vi "Autonomous Independent.vi"() -> ()   [LabVIEW 2016]
doc: "This VI is called when autonomous begins, and will automatically be terminated when autonomous ends. You can carry out timed or sensor driven robot movement independently without needing to return to the caller."
uses:
  <vilib>/Rock Robotics/WPI/ThirdParty/CanMotor/TalonSRX/WPI_CANTalonSRX_APIControlMode.ctl
  <vilib>/Rock Robotics/WPI/DriverStation/WPI_DriverStationAllianceInfo.ctl
  <vilib>/Rock Robotics/Network Tables/NT Read Boolean.vi
  Robot Global Data.vi
panel:
  out "Auto time":u32
  # "Be sure to right-click and choose Data Operations>>Make Current Value default if you want to save the array values with the VI"
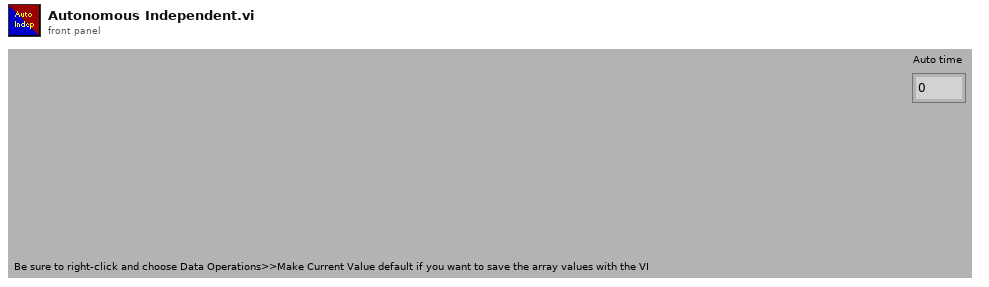
[diagram p1: front panel]
types:
  T1 = typedef "WPI_DriverStationAllianceInfo.ctl" = enum16{"Red", "Blue", "Invalid"}
  T2 = typedef "WPI_CANTalonSRX_APIControlMode.ctl" = enum8{"Percent VBus", "Speed", "Position", "Slave", "Unchanged / Invalid", "Voltage Compensation", "Current", "Motion Profile", "Motion Magic"}
  T3 = typedef "WPI_MotorControlDeviceRef.ctl" = cluster{"DeviceStatus":errorcluster, "Type":T4, "PWM":cluster{"PWM Channel":T5, "DeadBand":T6}, "CAN":cluster{"Device Number":u8, "SetOutput VI Ref":variant, "GetOutput VI Ref":variant, "Enable VI Ref":variant, "Disable VI Ref":variant, "Data":variant}, "Invert":bool}
  T4 = typedef "WPI_MotorControlType.ctl" = enum16{"PWM", "CAN"}
  T5 = typedef "FPGA_DIOPWMChannel.ctl" = enum8{"PWM 0", "PWM 1", "PWM 2", "PWM 3", "PWM 4", "PWM 5", "PWM 6", "PWM 7", "PWM 8", "PWM 9", "PWM MXP 0", "PWM MXP 1", "PWM MXP 2", "PWM MXP 3", "PWM MXP 4", "PWM MXP 5", "PWM MXP 6", "PWM MXP 7", "PWM MXP 8", "PWM MXP 9", "Invalid"}
  T6 = typedef "WPI_PWMDeadband.ctl" = cluster{"Name":string, "maxPositivePwm":i32, "minPositivePwm":i32, "centerPwm":i32, "maxNegativePwm":i32, "minNegativePwm":i32, "angularRange":u16}
  T7 = cluster{"Yaw":dbl, "Roll":dbl, "Pitch":dbl, "Heading":dbl, "Fused Heading":dbl}
  T8 = typedef "WPI_CANTalonSRX_GlobalStatus.ctl" = cluster{"Applied Throttle":dbl, "Module Enabled":bool, "CAN Error":errorcluster, "Closed Loop Error":dbl, "Forward Limit Switch Closed":bool, "Reverse Limit Switch Closed":bool, "Sensor Position":dbl, "Sensor Velocity":dbl, "Current":dbl, "Sticky Fault - Over Temp":bool, "Sticky Fault - Under Voltage":bool, "Sticky Fault - Forward Limit":bool, "Sticky Fault - Reverse Limit":bool, "Sticky Fault - Forward Soft Limit":bool, "Sticky Fault - Reverse Soft Limit":bool, "Brake is Enabled":bool, "Encoder Position":dbl, "Encoder Velocity":dbl, "Encoder Index Count":dbl, "Encoder A Pin State":bool, "Encoder B Pin State":bool, "Encoder Index Pin State":bool, "Analog In":dbl, "Analog In Velocity":dbl, "Temperature (C)":dbl, "Battery Voltage":dbl, "Control 5 Is Supported":bool, "Current Profile Slot Select":dbl, "Pos Div 8":bool, "Vel Div 4":bool, "Pulse Width Position":i32, "Pulse Width Velocity":i32, "Pulse Width Rise To Rise (us)":i32, "Pulse Width Rise To Fall (us)":i32, "Mot Prof Active Is Under Run":bool, "Mot Prof Active Has Under Run":bool, "Mot Prof Active Is Last":bool, "Mot Prof Active Velocity Only":bool, "Mot Prof Active Is Valid":bool, "Mot Prof Buffer Is Full":bool, "Mot Prof Active Profile Slot Select":i32, "Mot Prof NextID":i32, "Mot Prof Count":i32, "Mot Prof Active Velocity":dbl, "Mot Prof Active Position":dbl, "Mot Prof Output Enable":i32}
  T9 = cluster{"proportional gain (Kc)":dbl, "integral time (Ti, min)":dbl, "derivative time (Td, min)":dbl}
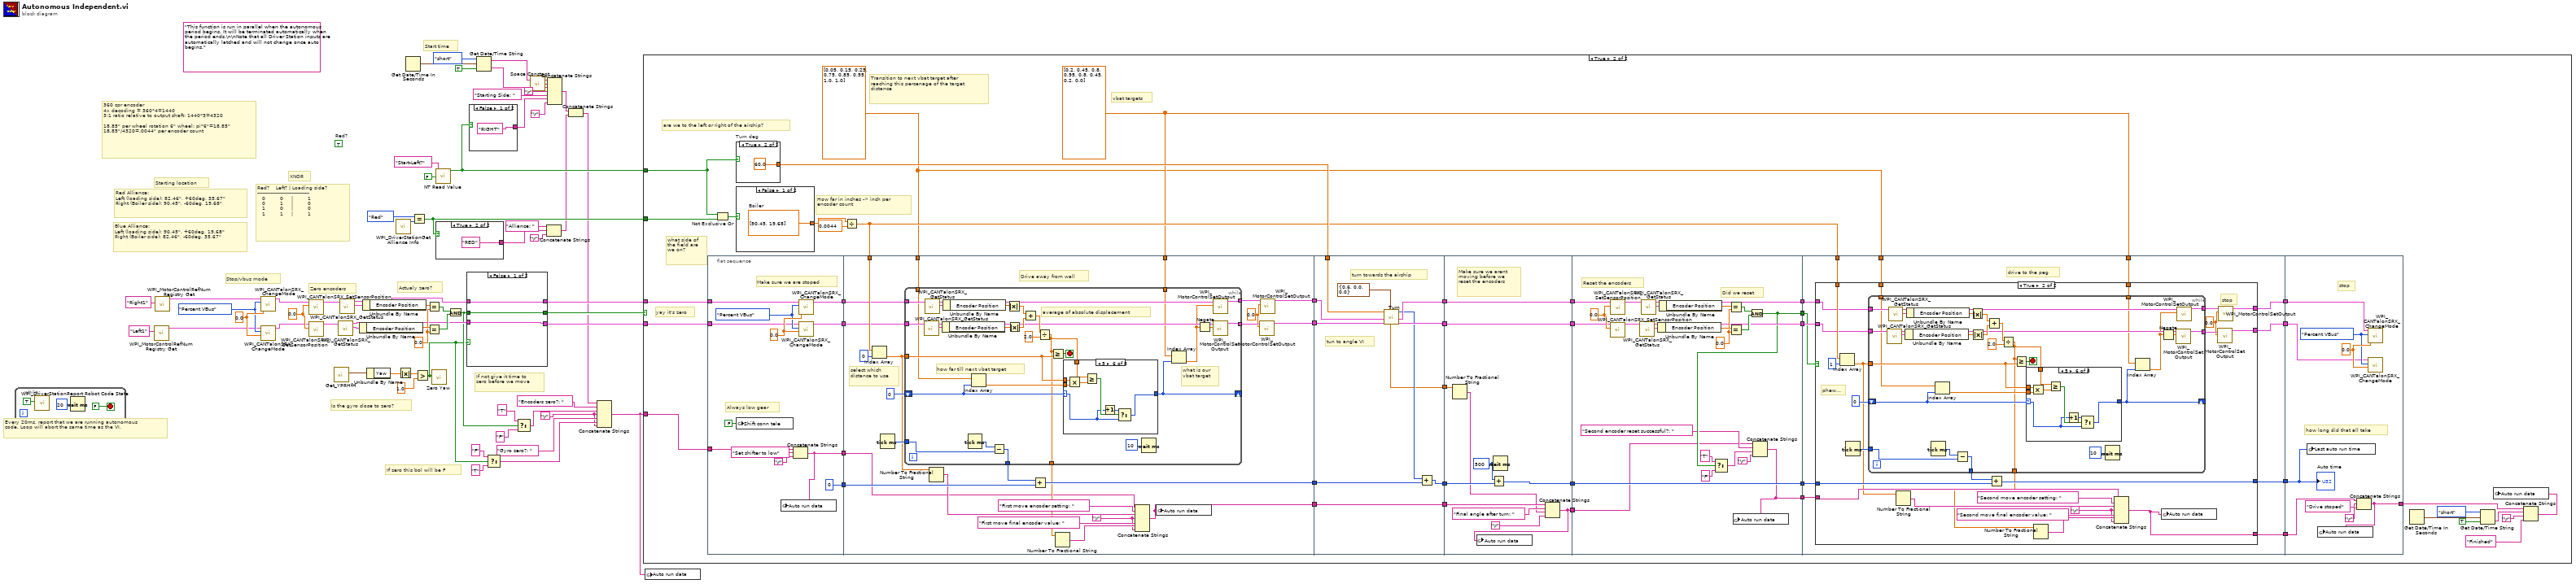
[diagram p0: block diagram]
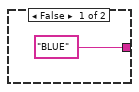
[diagram p2: hidden frame]
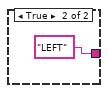
[diagram p3: hidden frame]
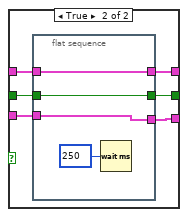
[diagram p4: hidden frame]
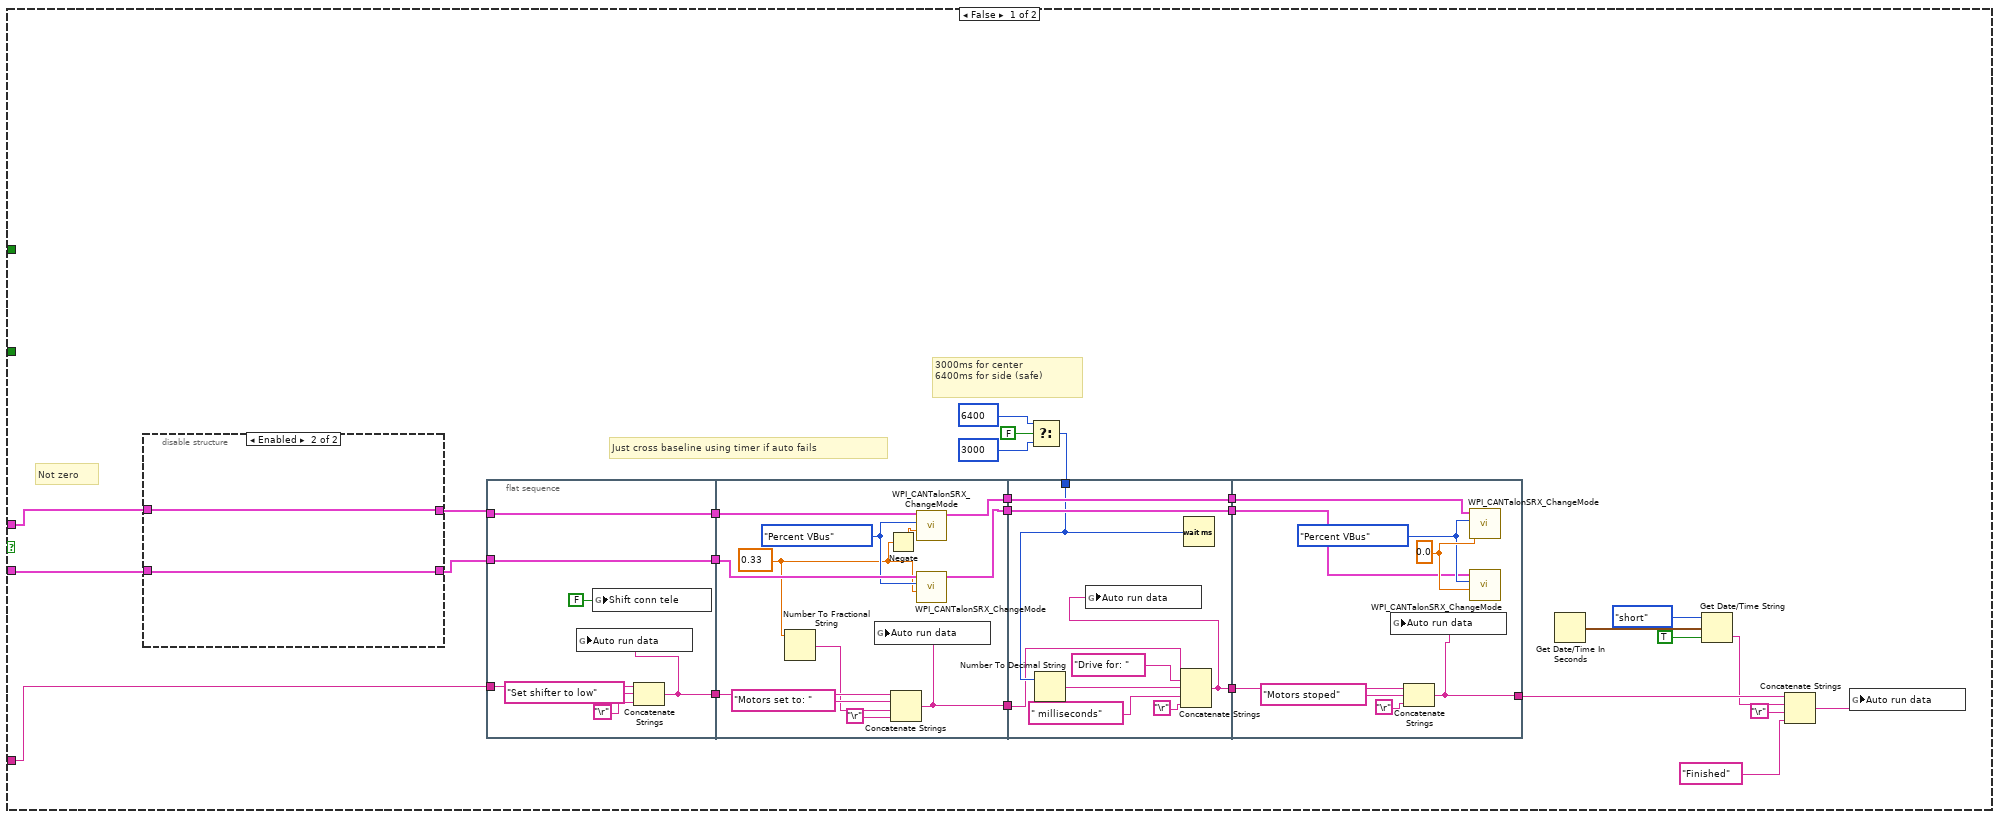
[diagram p5: hidden frame]
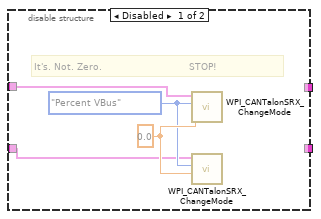
[diagram p6: hidden frame]
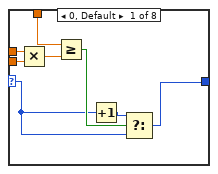
[diagram p7: hidden frame]
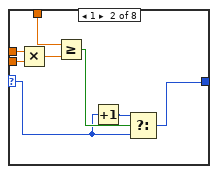
[diagram p8: hidden frame]
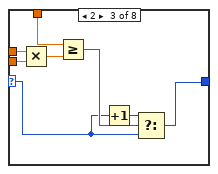
[diagram p9: hidden frame]
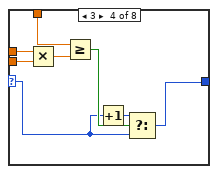
[diagram p10: hidden frame]
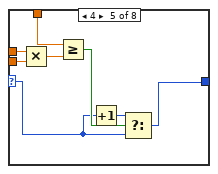
[diagram p11: hidden frame]
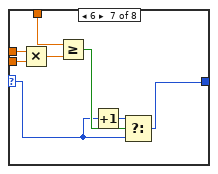
[diagram p12: hidden frame]
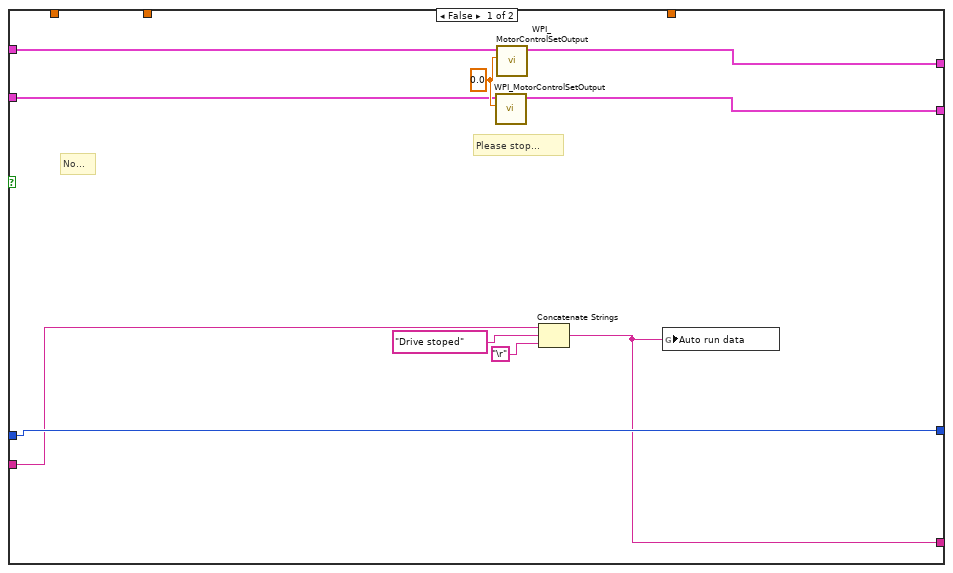
[diagram p14: hidden frame]
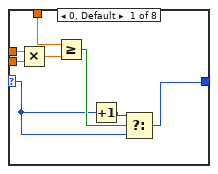
[diagram p15: hidden frame]
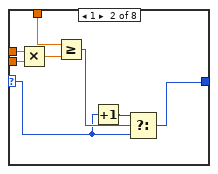
[diagram p16: hidden frame]
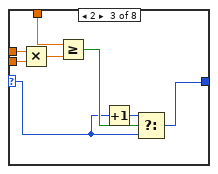
[diagram p17: hidden frame]
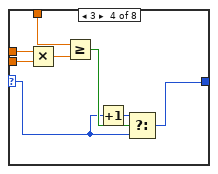
[diagram p18: hidden frame]
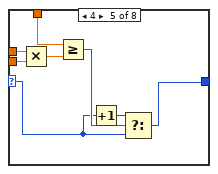
[diagram p19: hidden frame]
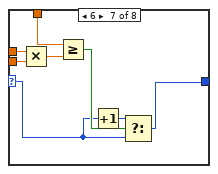
[diagram p20: hidden frame]
diagram:
  w9 = "\r"
  w40 = WPI_CANTalonSRX_APIControlMode."Percent VBus" ("Control Mode")
  w41 = 0.0
  w52 = 0.0
  w59 = 0.0 ("New Sensor Position")
  (unwired) TRUE  # Red?
  (unwired) "This function is run in parallel when the autonomous period begins. It will be terminated automatically when the period ends.\n\nNote that all Driver Station inputs are automatically latched and will not change once auto begins."
  # "Start time"
  # "If zero this bol will be F"
  # "Starting location"
  # "If not give it time to\nzero before we move"
  # "Is the gyro close to zero?"
  # "Stop/vbus mode"
  # "Zero encoders"
  # "Actualy zero?"
  # "XNOR"
  # "Red?    Left? | Loading side?\n--------------------------------\n   0         0     |         1        \n   0         1     |         0\n   1         0     |         0\n   1         1     |         1"
  # "Blue Alliance:\nLeft (loading side): 90.45\", +60deg, 19.68\"\nRight (Boiler side): 82.46\", -60deg, 35.67\""
  # "Red Alliance:\nLeft (loading side): 82.46\", +60deg, 35.67\"\nRight (Boiler side): 90.45\", -60deg, 19.68\""
  # "360 cpr encoder\n4x decoding = 360*4=1440\n3:1 ratio relative to output shaft: 1440*3=4320\n\n18.85\" per wheel rotation 6\" wheel: pi*6\"=18.85\"\n18.85\"/4320=.0044\" per encoder count"
  # "Every 20ms, report that we are running autonomous\ncode. Loop will abort the same time as the VI."
  n1 = while {
    stop <- FALSE stop-if-true
    n2 = call <vilib>:"WPI_DriverStationReport Robot Code State.vi"("Autonomous"=TRUE) -> ()  [unwired: 10 in, 1 out]
    n3 = Wait (ms)(milliseconds to wait=u32 20) -> ()  [unwired: 1 out]
  }
  n4 = call <vilib>:"WPI_MotorControlRefNum Registry Get.vi"("refnum name"="Left1") -> ("MotorControlDevRef"=w38:T3)  [unwired: 9 in, 1 out]
  n5 = call <vilib>:"WPI_MotorControlRefNum Registry Get.vi"("refnum name"="Right1") -> ("MotorControlDevRef"=w39:T3)  [unwired: 9 in, 1 out]
  n6 = call <vilib>:"WPI_CANTalonSRX_ChangeMode.vi"("Output"=w41, "Control Mode"=w40, "CAN Talon SRX Ref"=w39) -> ("CAN Talon SRX Ref"=w37:T3)  [unwired: 7 in, 1 out]
  n7 = call <vilib>:"WPI_CANTalonSRX_ChangeMode.vi"("Output"=w41, "Control Mode"=w40, "CAN Talon SRX Ref"=w38) -> ("CAN Talon SRX Ref"=w36:T3)  [unwired: 7 in, 1 out]
  n8 = call <vilib>:"WPI_CANTalonSRX_SetSensorPosition.vi"("New Sensor Position"=w59, "CAN Talon SRX Ref"=w36) -> ("CAN Talon SRX Ref"=w55:T3)  [unwired: 8 in, 1 out]
  n9 = call <vilib>:"WPI_CANTalonSRX_SetSensorPosition.vi"("New Sensor Position"=w59, "CAN Talon SRX Ref"=w37) -> ("CAN Talon SRX Ref"=w56:T3)  [unwired: 8 in, 1 out]
  n10 = call <vilib>:"Get_YPRHfH.vi"() -> ("YRPHfH"=w49:T7)  [unwired: 11 in]
  n11 = call <vilib>:"WPI_CANTalonSRX_GetStatus.vi"("CAN Talon SRX Ref"=w55) -> ("Talon SRX Status"=w57:T8, "CAN Talon SRX Ref"=w42:T3)  [unwired: 8 in, 1 out]
  n12 = call <vilib>:"WPI_CANTalonSRX_GetStatus.vi"("CAN Talon SRX Ref"=w56) -> ("Talon SRX Status"=w58:T8, "CAN Talon SRX Ref"=w43:T3)  [unwired: 8 in, 1 out]
  n13 = Unbundle By Name(w57) -> ("Encoder Position"=w53:dbl)
  n14 = Unbundle By Name(w58) -> ("Encoder Position"=w54:dbl)
  n15 = Unbundle By Name(w49) -> ("Yaw"=w48:dbl)
  n16 = call <vilib>:"WPI_DriverStationGet Alliance Info.vi"() -> ("Alliance"=w25:T1)  [unwired: 11 out]
  n17 = Absolute Value(x=w48) -> (abs(x)=w33:dbl)
  n18 = Get Date/Time In Seconds() -> (seconds since 1Jan1904=w7:timestamp)
  n19 = Equal?(x=WPI_DriverStationAllianceInfo."Red" ("Alliance"), y=w25) -> (x = y?=w23:bool)
  n20 = Greater?(x=w33, y=1.0) -> (0:w29:bool)
  n21 = Equal?(x=w54, y=w52) -> (x = y?=w51:bool)
  n22 = Equal?(x=w53, y=w52) -> (x = y?=w50:bool)
  n23 = call <vilib>:"Zero Yaw.vi"("Zero"=w29) -> ()  [unwired: 11 in]
  n24 = call-poly <vilib>:"NT Read Value.vi"("Default Value"=FALSE, "Name"="Start-Left?") -> ("Boolean"=w24:bool)  [unwired: 8 in, 1 out]
  n25 = case shown="True" w23 {
    tunnel: ["BLUE" "RED"] -> w21
    frame False {
    }
    frame True {
    }
  }
  n26 = And(x=w51, y=w50) -> (x .and. y?=w30:bool)
  n27 = case shown="False" w29 {
    tunnel: [w68 w75] -> w46
    tunnel: [w67 w71] -> w45
    tunnel: w30 -> [w69 w72]
    tunnel: [w69 w73] -> w44
    tunnel: w43 -> [w68 w74]
    tunnel: w42 -> [w67 w70]
    frame False {
    }
    frame True {
      n28 = flat-sequence {
        tunnel: [w79] -> w75
        tunnel: w74 -> [w79]
        tunnel: [w78] -> w73
        tunnel: w72 -> [w78]
        tunnel: [w77] -> w71
        tunnel: w70 -> [w77]
        frame #0 {
          n29 = Wait (ms)(milliseconds to wait=u32 250) -> ()  [unwired: 1 out]
        }
      }
    }
  }
  n30 = case shown="False" w24 {
    tunnel: ["RIGHT" "LEFT"] -> w17
    frame False {
    }
    frame True {
    }
  }
  n31 = Get Date/Time String(date format (0)=enum16{"short", "long", "abbreviated"}."short", seconds (now)=w7, want seconds? (F)=TRUE) -> (date string=w3:string, time string=w2:string)
  n32 = Select(t="F", s=w29, f="T") -> (s? t:f=w10:string)
  n33 = Select(t="T", s=w30, f="F") -> (s? t:f=w12:string)
  n34 = call <vilib>:"Space Constant.vi"() -> ("String"=w1:string)
  n35 = Concatenate Strings("Alliance: ", w21, "\r") -> (w15:string)
  n36 = Concatenate Strings(w3, w1, w2, "\r", "Starting Side: ", w17, "\r") -> (w16:string)
  n37 = Concatenate Strings(w16, w15) -> (w14:string)
  n38 = Concatenate Strings(w14, "Encoders zero?: ", w12, w9, "Gyro zero?: ", w10, w9) -> (w8:string)
  n39 = case shown="True" w44 {
    tunnel: w46 -> [w107 w181]
    tunnel: w45 -> [w106 w180]
    tunnel: w24 -> [_ w167]
    tunnel: w23 -> [_ w166]
    tunnel: w8 -> [w97 w165]
    frame False {
      # "3000ms for center\n6400ms for side (safe)"
      # "Not zero"
      # "Just cross baseline using timer if auto fails"
      n40 = disable-structure shown="Enabled" {
        disable-tunnel: w107 -> [w145 w149]
        disable-tunnel: w106 -> [w144 w148]
        disable-tunnel: [_ w149] -> w99
        disable-tunnel: [_ w148] -> w98
        frame Disabled {
          w146 = WPI_CANTalonSRX_APIControlMode."Percent VBus" ("Control Mode")
          w147 = 0.0
          # "It's. Not. Zero.                             STOP!"
          n41 = call <vilib>:"WPI_CANTalonSRX_ChangeMode.vi"("Output"=w147, "Control Mode"=w146, "CAN Talon SRX Ref"=w145) -> ()  [unwired: 7 in, 2 out]
          n42 = call <vilib>:"WPI_CANTalonSRX_ChangeMode.vi"("Output"=w147, "Control Mode"=w146, "CAN Talon SRX Ref"=w144) -> ()  [unwired: 7 in, 2 out]
        }
        frame Enabled {
        }
      }
      n43 = flat-sequence {
        tunnel: w98 -> [w113]
        tunnel: w99 -> [w114]
        tunnel: [w114] -> w105
        tunnel: [w113] -> w104
        tunnel: w97 -> [w111]
        tunnel: [w108] -> w96
        tunnel: [w124] -> w103
        tunnel: [w123] -> w102
        tunnel: w105 -> [w126]
        tunnel: w104 -> [w125]
        tunnel: w96 -> [w120]
        tunnel: [w115] -> w95
        tunnel: w103 -> [w135]
        tunnel: w102 -> [w134]
        tunnel: [w135] -> w101
        tunnel: [w134] -> w100
        tunnel: w95 -> [w129]
        tunnel: w92 -> [w133]
        tunnel: [w127] -> w91
        tunnel: w101 -> [w141]
        tunnel: w100 -> [w140]
        tunnel: w91 -> [w139]
        tunnel: [w136] -> w90
        frame #0 {
          n44 = global write "Robot Global Data.vi" "Shift conn tele"(FALSE ("Shift conn tele")) -> ()
          n45 = Concatenate Strings(w111, "Set shifter to low" ("string"), "\r") -> (w108:string)
          n46 = global write "Robot Global Data.vi" "Auto run data"(w108) -> ()
        }
        frame #1 {
          w119 = 0.33 ("Output")
          w122 = WPI_CANTalonSRX_APIControlMode."Percent VBus" ("Control Mode")
          n47 = Number To Fractional String(number=w119) -> (F-format string=w117:string)  [unwired: 3 in]
          n48 = Negate(x=w119) -> (-x=w121:dbl)
          n49 = Concatenate Strings(w120, "Motors set to: ", w117, "\r") -> (w115:string)
          n50 = global write "Robot Global Data.vi" "Auto run data"(w115) -> ()
          n51 = call <vilib>:"WPI_CANTalonSRX_ChangeMode.vi"("Output"=w121, "Control Mode"=w122, "CAN Talon SRX Ref"=w126) -> ("CAN Talon SRX Ref"=w124:T3)  [unwired: 7 in, 1 out]
          n52 = call <vilib>:"WPI_CANTalonSRX_ChangeMode.vi"("Output"=w119, "Control Mode"=w122, "CAN Talon SRX Ref"=w125) -> ("CAN Talon SRX Ref"=w123:T3)  [unwired: 7 in, 1 out]
        }
        frame #2 {
          n53 = Number To Decimal String(number=w133) -> (decimal integer string=w131:string)  [unwired: 1 in]
          n54 = Concatenate Strings(w129, "Drive for: ", w131, " milliseconds", "\r") -> (w127:string)
          n55 = global write "Robot Global Data.vi" "Auto run data"(w127) -> ()
          n56 = Wait (ms)(milliseconds to wait=w133) -> ()  [unwired: 1 out]
        }
        frame #3 {
          w142 = WPI_CANTalonSRX_APIControlMode."Percent VBus" ("Control Mode")
          w143 = 0.0
          n57 = Concatenate Strings(w139, "Motors stoped" ("string"), "\r") -> (w136:string)
          n58 = global write "Robot Global Data.vi" "Auto run data"(w136) -> ()
          n59 = call <vilib>:"WPI_CANTalonSRX_ChangeMode.vi"("Output"=w143, "Control Mode"=w142, "CAN Talon SRX Ref"=w141) -> ()  [unwired: 7 in, 2 out]
          n60 = call <vilib>:"WPI_CANTalonSRX_ChangeMode.vi"("Output"=w143, "Control Mode"=w142, "CAN Talon SRX Ref"=w140) -> ()  [unwired: 7 in, 2 out]
        }
      }
      n61 = Select(t=u32 6400 ("milliseconds to wait"), s=FALSE, f=u32 3000 ("milliseconds to wait")) -> (s? t:f=w92:u32)
      n62 = Get Date/Time In Seconds() -> (seconds since 1Jan1904=w87:timestamp)
      n63 = Get Date/Time String(date format (0)=enum16{"short", "long", "abbreviated"}."short", seconds (now)=w87, want seconds? (F)=TRUE) -> (time string=w84:string)  [unwired: 1 out]
      n64 = Concatenate Strings(w90, w84, "\r", "Finished") -> (w89:string)
      n65 = global write "Robot Global Data.vi" "Auto run data"(w89) -> ()
    }
    frame True {
      w178 = dbl[] [0.05, 0.15, 0.25, 0.75, 0.85, 0.95, 1.0, 1.0]
      w179 = dbl[] [0.2, 0.45, 0.8, 0.95, 0.8, 0.45, 0.2, 0.0]
      # "vbat targets"
      # "How far in inches -> inch per \nencoder count"
      # "Transition to next vbat target after\nreaching this percenage of the target\ndistance"
      # "are we to the left or right of the airship?"
      # "what side of\nthe field are\nwe on?"
      # "yay it's zero"
      n66 = flat-sequence {
        tunnel: w181 -> [w203]
        tunnel: w180 -> [w201]
        tunnel: [w200] -> w195
        tunnel: [w202] -> w194
        tunnel: [u32 0 ("Turn time out")] -> w193
        tunnel: w165 -> [w197]
        tunnel: [w196] -> w161
        tunnel: w195 -> [w227]
        tunnel: w194 -> [w228]
        tunnel: w182 -> [w232]
        tunnel: [w230] -> w192
        tunnel: w193 -> [w229]
        tunnel: [w220] -> w191
        tunnel: [w218] -> w190
        tunnel: w179 -> [w224]
        tunnel: w178 -> [w222]
        tunnel: [w209] -> w163
        tunnel: w161 -> [w208]
        tunnel: w185 -> [w320]
        tunnel: [w325] -> w173
        tunnel: [w324] -> w171
        tunnel: w192 -> [w322]
        tunnel: [w321] -> w169
        tunnel: w191 -> [w327]
        tunnel: w190 -> [w326]
        tunnel: [w319] -> w164
        tunnel: w163 -> [w318]
        tunnel: [w318] -> w162
        tunnel: w173 -> [w339]
        tunnel: [w339] -> w172
        tunnel: w171 -> [w338]
        tunnel: [w338] -> w170
        tunnel: w169 -> [w337]
        tunnel: [w336] -> w168
        tunnel: w164 -> [w334]
        tunnel: w162 -> [w333]
        tunnel: [w329] -> w160
        tunnel: w172 -> [w351]
        tunnel: [w349] -> w177
        tunnel: w170 -> [w350]
        tunnel: [w348] -> w176
        tunnel: w168 -> [w362]
        tunnel: [w362] -> w175
        tunnel: [w345] -> w174
        tunnel: w160 -> [w343]
        tunnel: [w342] -> w159
        tunnel: w177 -> [w369]
        tunnel: w182 -> [w374]
        tunnel: [w370] -> w189
        tunnel: [w371] -> w188
        tunnel: w176 -> [w368]
        tunnel: w175 -> [w373]
        tunnel: [w372] -> w187
        tunnel: w179 -> [w367]
        tunnel: w178 -> [w366]
        tunnel: w174 -> [w365]
        tunnel: w159 -> [w364]
        tunnel: [w363] -> w158
        tunnel: w189 -> [w500]
        tunnel: w188 -> [w501]
        tunnel: w187 -> [w499]
        tunnel: w158 -> [w496]
        tunnel: [w495] -> w154
        frame #0 {
          w204 = WPI_CANTalonSRX_APIControlMode."Percent VBus" ("Control Mode")
          w205 = 0.0
          # "Always low gear"
          # "Make sure we are stoped"
          n67 = global write "Robot Global Data.vi" "Shift conn tele"(FALSE ("Shift conn tele")) -> ()
          n68 = Concatenate Strings(w197, "Set shifter to low" ("string"), "\r") -> (w196:string)
          n69 = global write "Robot Global Data.vi" "Auto run data"(w196) -> ()
          n70 = call <vilib>:"WPI_CANTalonSRX_ChangeMode.vi"("Output"=w205, "Control Mode"=w204, "CAN Talon SRX Ref"=w203) -> ("CAN Talon SRX Ref"=w202:T3)  [unwired: 7 in, 1 out]
          n71 = call <vilib>:"WPI_CANTalonSRX_ChangeMode.vi"("Output"=w205, "Control Mode"=w204, "CAN Talon SRX Ref"=w201) -> ("CAN Talon SRX Ref"=w200:T3)  [unwired: 7 in, 1 out]
        }
        frame #1 {
          w210 = "\r"
          w217 = 0.0
          # "select which\ndistance to use"
          # "Drive away from wall"
          n72 = Index Array(array=w232, index=0) -> (element=w213:dbl)
          n73 = Tick Count (ms)() -> (millisecond timer value=w226:u32)
          n74 = while {
            tunnel: w228 -> [w251]
            tunnel: w227 -> [w250]
            tunnel: [w247] -> w221
            tunnel: [w246] -> w219
            tunnel: w213 -> [w238]
            tunnel: w226 -> [w242]
            tunnel: [w243] -> w225
            tunnel: w224 -> [w241]
            shift-right: [w237] -> _
            shift-left: u8 0 -> [w236]
            tunnel: w222 -> [w235]
            tunnel: [w233] -> w214
            stop <- w260 stop-if-true
            # "what is our\nvbat target"
            # "how far till next vbat target"
            # "average of absolute displacement"
            n75 = call <vilib>:"WPI_CANTalonSRX_GetStatus.vi"("CAN Talon SRX Ref"=w250) -> ("Talon SRX Status"=w253:T8, "CAN Talon SRX Ref"=w248:T3)  [unwired: 8 in, 1 out]
            n76 = call <vilib>:"WPI_CANTalonSRX_GetStatus.vi"("CAN Talon SRX Ref"=w251) -> ("Talon SRX Status"=w252:T8, "CAN Talon SRX Ref"=w249:T3)  [unwired: 8 in, 1 out]
            n77 = Unbundle By Name(w253) -> ("Encoder Position"=w255:dbl)
            n78 = Unbundle By Name(w252) -> ("Encoder Position"=w254:dbl)
            n79 = Tick Count (ms)() -> (millisecond timer value=w244:u32)
            n80 = Index Array(array=w235, index=w236) -> (element=w234:dbl)
            n81 = Subtract(x=w244, y=w242) -> (x-y=w243:u32)
            n82 = Absolute Value(x=w254) -> (abs(x)=w256:dbl)
            n83 = Absolute Value(x=w255) -> (abs(x)=w257:dbl)
            n84 = Add(x=w256, y=w257) -> (x+y=w258:dbl)
            n85 = Divide(x=w258, y=2.0) -> (x/y=w233:dbl)
            n86 = Greater Or Equal?(x=w233, y=w238) -> (x >= y?=w260:bool)
            n87 = case shown="5" w236 {
              selector: w236 -> [w263 w270 w278 w286 w294 w302 w310 w317]
              tunnel: [w267 w275 w283 w291 w299 w307 w315 w317] -> w237
              tunnel: w233 -> [w265 w273 w281 w289 w297 w305 w313 _]
              tunnel: w238 -> [w268 w276 w284 w292 w300 w308 w316 _]
              tunnel: w234 -> [w261 w269 w277 w285 w293 w301 w309 _]
              frame 0, Default {
                n88 = Multiply(x=w268, y=w261) -> (x*y=w266:dbl)
                n89 = Greater Or Equal?(x=w265, y=w266) -> (x >= y?=w264:bool)
                n90 = Increment(x=w263) -> (x+1=w262:u8)
                n91 = Select(t=w262, s=w264, f=w263) -> (s? t:f=w267:u8)
              }
              frame 1 {
                n92 = Multiply(x=w276, y=w269) -> (x*y=w274:dbl)
                n93 = Greater Or Equal?(x=w273, y=w274) -> (x >= y?=w272:bool)
                n94 = Increment(x=w270) -> (x+1=w271:u8)
                n95 = Select(t=w271, s=w272, f=w270) -> (s? t:f=w275:u8)
              }
              frame 2 {
                n96 = Multiply(x=w284, y=w277) -> (x*y=w282:dbl)
                n97 = Greater Or Equal?(x=w281, y=w282) -> (x >= y?=w280:bool)
                n98 = Increment(x=w278) -> (x+1=w279:u8)
                n99 = Select(t=w279, s=w280, f=w278) -> (s? t:f=w283:u8)
              }
              frame 3 {
                n100 = Multiply(x=w292, y=w285) -> (x*y=w290:dbl)
                n101 = Greater Or Equal?(x=w289, y=w290) -> (x >= y?=w288:bool)
                n102 = Increment(x=w286) -> (x+1=w287:u8)
                n103 = Select(t=w287, s=w288, f=w286) -> (s? t:f=w291:u8)
              }
              frame 4 {
                n104 = Multiply(x=w300, y=w293) -> (x*y=w298:dbl)
                n105 = Greater Or Equal?(x=w297, y=w298) -> (x >= y?=w296:bool)
                n106 = Increment(x=w294) -> (x+1=w295:u8)
                n107 = Select(t=w295, s=w296, f=w294) -> (s? t:f=w299:u8)
              }
              frame 5 {
                n108 = Multiply(x=w308, y=w301) -> (x*y=w306:dbl)
                n109 = Greater Or Equal?(x=w305, y=w306) -> (x >= y?=w304:bool)
                n110 = Increment(x=w302) -> (x+1=w303:u8)
                n111 = Select(t=w303, s=w304, f=w302) -> (s? t:f=w307:u8)
              }
              frame 6 {
                n112 = Multiply(x=w316, y=w309) -> (x*y=w314:dbl)
                n113 = Greater Or Equal?(x=w313, y=w314) -> (x >= y?=w312:bool)
                n114 = Increment(x=w310) -> (x+1=w311:u8)
                n115 = Select(t=w311, s=w312, f=w310) -> (s? t:f=w315:u8)
              }
              frame 7 {
              }
            }
            n116 = Wait (ms)(milliseconds to wait=u32 10) -> ()  [unwired: 1 out]
            n117 = Index Array(array=w241, index=w237) -> (element=w240:dbl)
            n118 = Negate(x=w240) -> (-x=w239:dbl)
            n119 = call <vilib>:"WPI_MotorControlSetOutput.vi"("Output"=w239, "MotorControlDevRef"=w248) -> ("MotorControlDevRef"=w246:T3)  [unwired: 7 in, 2 out]
            n120 = call <vilib>:"WPI_MotorControlSetOutput.vi"("Output"=w240, "MotorControlDevRef"=w249) -> ("MotorControlDevRef"=w247:T3)  [unwired: 7 in, 2 out]
          }
          n121 = Number To Fractional String(number=w213) -> (F-format string=w215:string)  [unwired: 3 in]
          n122 = Add(x=w225, y=w229) -> (x+y=w230:u32)
          n123 = Number To Fractional String(number=w214) -> (F-format string=w211:string)  [unwired: 3 in]
          n124 = Concatenate Strings(w208, "First move encoder setting: ", w215, w210, "First move final encoder value: ", w211, w210) -> (w209:string)
          n125 = global write "Robot Global Data.vi" "Auto run data"(w209) -> ()
          n126 = call <vilib>:"WPI_MotorControlSetOutput.vi"("Output"=w217, "MotorControlDevRef"=w219) -> ("MotorControlDevRef"=w218:T3)  [unwired: 7 in, 2 out]
          n127 = call <vilib>:"WPI_MotorControlSetOutput.vi"("Output"=w217, "MotorControlDevRef"=w221) -> ("MotorControlDevRef"=w220:T3)  [unwired: 7 in, 2 out]
        }
        frame #2 {
          # "turn towards the airship"
          # "tun to angle VI"
          n128 = call "Turn.vi"("PID gains"=T9 {"proportional gain (Kc)"=0.6, "integral time (Ti, min)"=0.0, "derivative time (Td, min)"=0.0}, "Right MotorControlDevRef in"=w326, "Left MotorControlDevRef in"=w327, "Gyro target"=w320) -> ("Right MotorControlDevRef out"=w324:T3, "Left MotorControlDevRef out"=w325:T3, "Turn time out"=w323:u32, "Yaw out"=w319:dbl)  [unwired: 4 in]
          n129 = Add(x=w323, y=w322) -> (x+y=w321:u32)
        }
        frame #3 {
          w335 = u32 500 ("milliseconds to wait")
          # "Make sure we arent\nmoving before we\nreset the encoders"
          n130 = Number To Fractional String(number=w334) -> (F-format string=w331:string)  [unwired: 3 in]
          n131 = Add(x=w335, y=w337) -> (x+y=w336:u32)
          n132 = Wait (ms)(milliseconds to wait=w335) -> ()  [unwired: 1 out]
          n133 = Concatenate Strings(w333, "Final angle after turn: ", w331, "\r") -> (w329:string)
          n134 = global write "Robot Global Data.vi" "Auto run data"(w329) -> ()
        }
        frame #4 {
          w354 = 0.0
          w361 = 0.0 ("New Sensor Position")
          # "Did we reset"
          # "Reset the encoders"
          n135 = call <vilib>:"WPI_CANTalonSRX_SetSensorPosition.vi"("New Sensor Position"=w361, "CAN Talon SRX Ref"=w350) -> ("CAN Talon SRX Ref"=w357:T3)  [unwired: 8 in, 1 out]
          n136 = call <vilib>:"WPI_CANTalonSRX_SetSensorPosition.vi"("New Sensor Position"=w361, "CAN Talon SRX Ref"=w351) -> ("CAN Talon SRX Ref"=w358:T3)  [unwired: 8 in, 1 out]
          n137 = call <vilib>:"WPI_CANTalonSRX_GetStatus.vi"("CAN Talon SRX Ref"=w357) -> ("Talon SRX Status"=w359:T8, "CAN Talon SRX Ref"=w348:T3)  [unwired: 8 in, 1 out]
          n138 = call <vilib>:"WPI_CANTalonSRX_GetStatus.vi"("CAN Talon SRX Ref"=w358) -> ("Talon SRX Status"=w360:T8, "CAN Talon SRX Ref"=w349:T3)  [unwired: 8 in, 1 out]
          n139 = Unbundle By Name(w359) -> ("Encoder Position"=w355:dbl)
          n140 = Unbundle By Name(w360) -> ("Encoder Position"=w356:dbl)
          n141 = Equal?(x=w356, y=w354) -> (x = y?=w353:bool)
          n142 = Equal?(x=w355, y=w354) -> (x = y?=w352:bool)
          n143 = And(x=w353, y=w352) -> (x .and. y?=w345:bool)
          n144 = Select(t="T", s=w345, f="F") -> (s? t:f=w341:string)
          n145 = Concatenate Strings(w343, "Second encoder reset successful?: ", w341, "\r") -> (w342:string)
          n146 = global write "Robot Global Data.vi" "Auto run data"(w342) -> ()
        }
        frame #5 {
          # "drive to the peg"
          n147 = case shown="True" w365 {
            tunnel: w374 -> [_ w408]
            tunnel: w373 -> [w379 w407]
            tunnel: [w379 w406] -> w372
            tunnel: [w381 w402] -> w371
            tunnel: [w380 w401] -> w370
            tunnel: w369 -> [w383 w400]
            tunnel: w368 -> [w382 w399]
            tunnel: w367 -> [_ w395]
            tunnel: w366 -> [_ w394]
            tunnel: w364 -> [w378 w389]
            tunnel: [w377 w385] -> w363
            frame False {
              w384 = 0.0
              # "Please stop..."
              # "No..."
              n148 = call <vilib>:"WPI_MotorControlSetOutput.vi"("Output"=w384, "MotorControlDevRef"=w382) -> ("MotorControlDevRef"=w380:T3)  [unwired: 7 in, 2 out]
              n149 = call <vilib>:"WPI_MotorControlSetOutput.vi"("Output"=w384, "MotorControlDevRef"=w383) -> ("MotorControlDevRef"=w381:T3)  [unwired: 7 in, 2 out]
              n150 = Concatenate Strings(w378, "Drive stoped", "\r") -> (w377:string)
              n151 = global write "Robot Global Data.vi" "Auto run data"(w377) -> ()
            }
            frame True {
              w390 = "\r"
              w403 = 0.0
              # "stop"
              # "phew..."
              n152 = Index Array(array=w408, index=1) -> (element=w387:dbl)
              n153 = Tick Count (ms)() -> (millisecond timer value=w397:u32)
              n154 = while {
                tunnel: w400 -> [w428]
                tunnel: w399 -> [w427]
                tunnel: [w424] -> w405
                tunnel: [w423] -> w404
                tunnel: w387 -> [w415]
                tunnel: w397 -> [w419]
                tunnel: [w420] -> w396
                tunnel: w395 -> [w418]
                shift-right: [w414] -> _
                shift-left: u8 0 -> [w413]
                tunnel: w394 -> [w412]
                tunnel: [w410] -> w386
                stop <- w437 stop-if-true
                n155 = call <vilib>:"WPI_CANTalonSRX_GetStatus.vi"("CAN Talon SRX Ref"=w427) -> ("Talon SRX Status"=w430:T8, "CAN Talon SRX Ref"=w425:T3)  [unwired: 8 in, 1 out]
                n156 = call <vilib>:"WPI_CANTalonSRX_GetStatus.vi"("CAN Talon SRX Ref"=w428) -> ("Talon SRX Status"=w429:T8, "CAN Talon SRX Ref"=w426:T3)  [unwired: 8 in, 1 out]
                n157 = Unbundle By Name(w430) -> ("Encoder Position"=w432:dbl)
                n158 = Unbundle By Name(w429) -> ("Encoder Position"=w431:dbl)
                n159 = Tick Count (ms)() -> (millisecond timer value=w421:u32)
                n160 = Index Array(array=w412, index=w413) -> (element=w411:dbl)
                n161 = Subtract(x=w421, y=w419) -> (x-y=w420:u32)
                n162 = Absolute Value(x=w431) -> (abs(x)=w433:dbl)
                n163 = Absolute Value(x=w432) -> (abs(x)=w434:dbl)
                n164 = Add(x=w433, y=w434) -> (x+y=w435:dbl)
                n165 = Divide(x=w435, y=2.0) -> (x/y=w410:dbl)
                n166 = Greater Or Equal?(x=w410, y=w415) -> (x >= y?=w437:bool)
                n167 = case shown="5" w413 {
                  selector: w413 -> [w440 w447 w455 w463 w471 w479 w487 w494]
                  tunnel: [w444 w452 w460 w468 w476 w484 w492 w494] -> w414
                  tunnel: w410 -> [w442 w450 w458 w466 w474 w482 w490 _]
                  tunnel: w415 -> [w445 w453 w461 w469 w477 w485 w493 _]
                  tunnel: w411 -> [w438 w446 w454 w462 w470 w478 w486 _]
                  frame 0, Default {
                    n168 = Multiply(x=w445, y=w438) -> (x*y=w443:dbl)
                    n169 = Greater Or Equal?(x=w442, y=w443) -> (x >= y?=w441:bool)
                    n170 = Increment(x=w440) -> (x+1=w439:u8)
                    n171 = Select(t=w439, s=w441, f=w440) -> (s? t:f=w444:u8)
                  }
                  frame 1 {
                    n172 = Multiply(x=w453, y=w446) -> (x*y=w451:dbl)
                    n173 = Greater Or Equal?(x=w450, y=w451) -> (x >= y?=w449:bool)
                    n174 = Increment(x=w447) -> (x+1=w448:u8)
                    n175 = Select(t=w448, s=w449, f=w447) -> (s? t:f=w452:u8)
                  }
                  frame 2 {
                    n176 = Multiply(x=w461, y=w454) -> (x*y=w459:dbl)
                    n177 = Greater Or Equal?(x=w458, y=w459) -> (x >= y?=w457:bool)
                    n178 = Increment(x=w455) -> (x+1=w456:u8)
                    n179 = Select(t=w456, s=w457, f=w455) -> (s? t:f=w460:u8)
                  }
                  frame 3 {
                    n180 = Multiply(x=w469, y=w462) -> (x*y=w467:dbl)
                    n181 = Greater Or Equal?(x=w466, y=w467) -> (x >= y?=w465:bool)
                    n182 = Increment(x=w463) -> (x+1=w464:u8)
                    n183 = Select(t=w464, s=w465, f=w463) -> (s? t:f=w468:u8)
                  }
                  frame 4 {
                    n184 = Multiply(x=w477, y=w470) -> (x*y=w475:dbl)
                    n185 = Greater Or Equal?(x=w474, y=w475) -> (x >= y?=w473:bool)
                    n186 = Increment(x=w471) -> (x+1=w472:u8)
                    n187 = Select(t=w472, s=w473, f=w471) -> (s? t:f=w476:u8)
                  }
                  frame 5 {
                    n188 = Multiply(x=w485, y=w478) -> (x*y=w483:dbl)
                    n189 = Greater Or Equal?(x=w482, y=w483) -> (x >= y?=w481:bool)
                    n190 = Increment(x=w479) -> (x+1=w480:u8)
                    n191 = Select(t=w480, s=w481, f=w479) -> (s? t:f=w484:u8)
                  }
                  frame 6 {
                    n192 = Multiply(x=w493, y=w486) -> (x*y=w491:dbl)
                    n193 = Greater Or Equal?(x=w490, y=w491) -> (x >= y?=w489:bool)
                    n194 = Increment(x=w487) -> (x+1=w488:u8)
                    n195 = Select(t=w488, s=w489, f=w487) -> (s? t:f=w492:u8)
                  }
                  frame 7 {
                  }
                }
                n196 = Wait (ms)(milliseconds to wait=u32 10) -> ()  [unwired: 1 out]
                n197 = Index Array(array=w418, index=w414) -> (element=w417:dbl)
                n198 = Negate(x=w417) -> (-x=w416:dbl)
                n199 = call <vilib>:"WPI_MotorControlSetOutput.vi"("Output"=w416, "MotorControlDevRef"=w425) -> ("MotorControlDevRef"=w423:T3)  [unwired: 7 in, 2 out]
                n200 = call <vilib>:"WPI_MotorControlSetOutput.vi"("Output"=w417, "MotorControlDevRef"=w426) -> ("MotorControlDevRef"=w424:T3)  [unwired: 7 in, 2 out]
              }
              n201 = Number To Fractional String(number=w387) -> (F-format string=w388:string)  [unwired: 3 in]
              n202 = Add(x=w396, y=w407) -> (x+y=w406:u32)
              n203 = Number To Fractional String(number=w386) -> (F-format string=w391:string)  [unwired: 3 in]
              n204 = Concatenate Strings(w389, "Second move encoder setting: ", w388, w390, "Second move final encoder value: ", w391, w390) -> (w385:string)
              n205 = global write "Robot Global Data.vi" "Auto run data"(w385) -> ()
              n206 = call <vilib>:"WPI_MotorControlSetOutput.vi"("Output"=w403, "MotorControlDevRef"=w404) -> ("MotorControlDevRef"=w401:T3)  [unwired: 7 in, 2 out]
              n207 = call <vilib>:"WPI_MotorControlSetOutput.vi"("Output"=w403, "MotorControlDevRef"=w405) -> ("MotorControlDevRef"=w402:T3)  [unwired: 7 in, 2 out]
            }
          }
        }
        frame #6 {
          w502 = WPI_CANTalonSRX_APIControlMode."Percent VBus" ("Control Mode")
          w503 = 0.0
          # "how long did that all take"
          # "stop"
          n208 = global write "Robot Global Data.vi" "Last auto run time"(w499) -> ()
          n209 = Concatenate Strings(w496, "Drive stoped", "\r") -> (w495:string)
          n210 = global write "Robot Global Data.vi" "Auto run data"(w495) -> ()
          n211 = call <vilib>:"WPI_CANTalonSRX_ChangeMode.vi"("Output"=w503, "Control Mode"=w502, "CAN Talon SRX Ref"=w501) -> ()  [unwired: 7 in, 2 out]
          n212 = call <vilib>:"WPI_CANTalonSRX_ChangeMode.vi"("Output"=w503, "Control Mode"=w502, "CAN Talon SRX Ref"=w500) -> ()  [unwired: 7 in, 2 out]
          "Auto time" <- w499
        }
      }
      n213 = Not Exclusive Or(1:w166, 2:w167) -> (0:w186:bool)
      n214 = case "Turn deg" shown="True" w167 {
        tunnel: [-60.0 60.0] -> w185
        frame False {
        }
        frame True {
        }
      }
      n215 = case shown="False" w186 {
        tunnel: [w504 w505] -> w184
        frame False {
          w504 = dbl[] [90.45, 19.68]  # Boiler
        }
        frame True {
          w505 = dbl[] [82.46, 35.67]  # loading
        }
      }
      n216 = Divide(x=w184, y=0.0044) -> (x/y=w182:dbl[])
      n217 = Get Date/Time In Seconds() -> (seconds since 1Jan1904=w157:timestamp)
      n218 = Get Date/Time String(date format (0)=enum16{"short", "long", "abbreviated"}."short", seconds (now)=w157, want seconds? (F)=TRUE) -> (time string=w152:string)  [unwired: 1 out]
      n219 = Concatenate Strings(w154, w152, "\r", "Finished") -> (w153:string)
      n220 = global write "Robot Global Data.vi" "Auto run data"(w153) -> ()
    }
  }
  n221 = global write "Robot Global Data.vi" "Auto run data"(w8) -> ()
